vi "newChirp2oldChirpconversion.vi"(10 "scanVariables":dbl[][](array[numeric]), 11 "Chirp Parameters":T1) -> (3 "ChirpParameters":T2 {"miniscantime" format="%#_6e"})   [LabVIEW 2013]
uses:
  Controls/Chirp Parameters.ctl
panel:
  # "RE-ENTRANT"
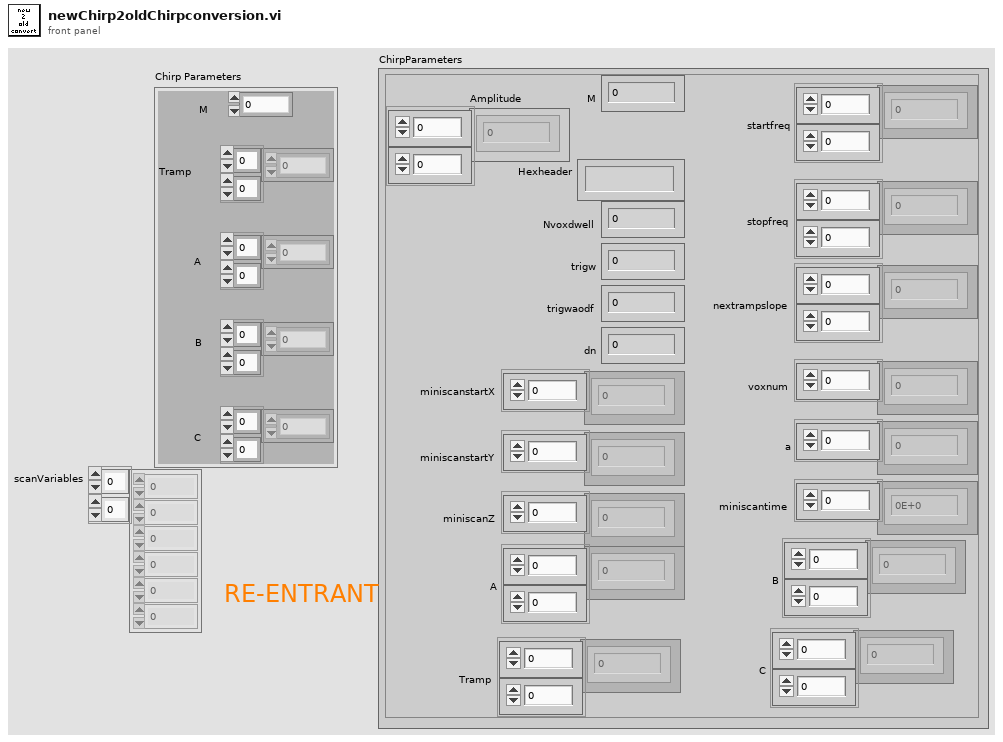
[diagram p1: front panel]
types:
  T1 = cluster{"M ":dbl, "Tramp":dbl[][], "A":dbl[][], "B":dbl[][], "C":dbl[][]}
  T2 = typedef "Chirp Parameters.ctl" = cluster{"M":dbl, "miniscantime":dbl[], "startfreq":dbl[][], "stopfreq":dbl[][], "nextrampslope":dbl[][], "Hexheader":string, "voxnum":dbl[], "Nvoxdwell":dbl, "miniscanstartX":dbl[], "miniscanstartY":dbl[], "miniscanZ":dbl[], "trigw":dbl, "trigwaodf":dbl, "dn":dbl, "a":dbl[], "A":dbl[][], "B":dbl[][], "Tramp":dbl[][], "C":dbl[][], "Amplitude":dbl[][]}
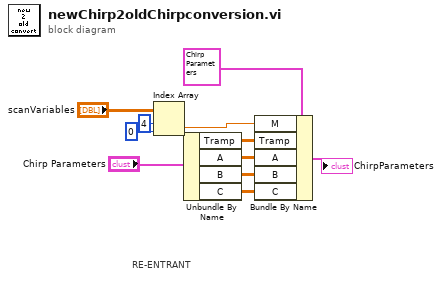
[diagram p0: block diagram]
diagram:
  # "RE-ENTRANT"
  n1 = Index Array(array="scanVariables", index (row)=4 ("index"), index (col)=0 ("disabled index (col)")) -> (element=w2:dbl)
  n2 = Unbundle By Name("Chirp Parameters") -> ("Tramp"=w8:dbl[][], "A"=w7:dbl[][], "B"=w6:dbl[][], "C"=w5:dbl[][])
  n3 = Bundle By Name(cluster=T2 {"M"=0.0, "miniscantime"=[], "startfreq"=[], "stopfreq"=[], "nextrampslope"=[], "Hexheader"="", "voxnum"=[], "Nvoxdwell"=0.0, "miniscanstartX"=[], "miniscanstartY"=[], "miniscanZ"=[], "trigw"=0.0, "trigwaodf"=0.0, "dn"=0.0, "a"=[], "A"=[], "B"=[], "Tramp"=[], "C"=[], "Amplitude"=[]} ("Chirp Parameters"), "M"=w2, "Tramp"=w8, "A"=w7, "B"=w6, "C"=w5) -> (→"ChirpParameters":T2)
